vi "Step Parser.vi"(0 "Profile Step":dbl[](array[numeric]), 11 "Brushed?":bool) -> (2 "VPIpara":i32, 4 "VoltPI":dbl format="%#_13g", 6 "PPIpara":i32, 8 "PresPI":dbl format="%#_13g", 10 "CPIpara":i32, 13 "Deadhead?":bool, 15 "CmdPI":dbl format="%#_13g")   [LabVIEW 2013]
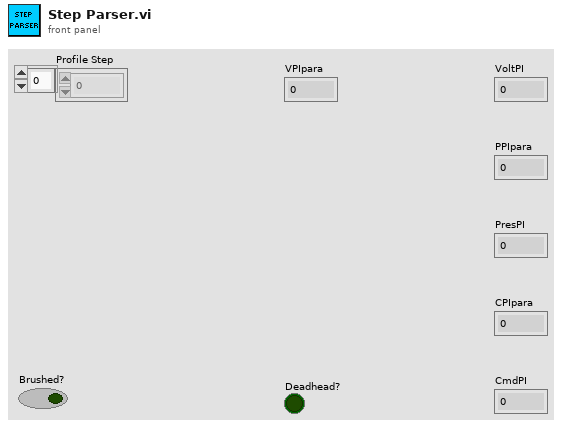
[diagram p1: front panel]
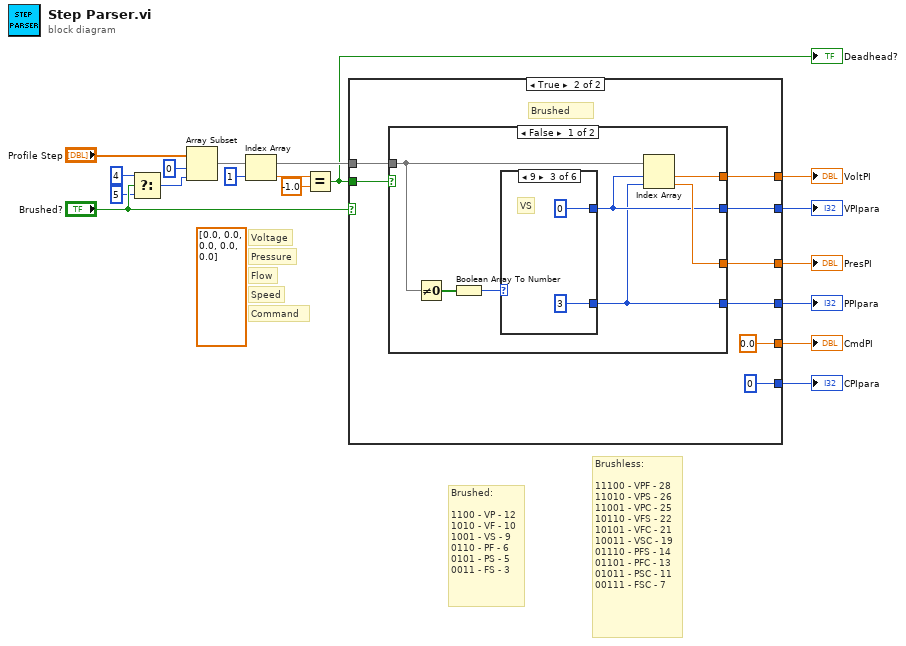
[diagram p0: block diagram]
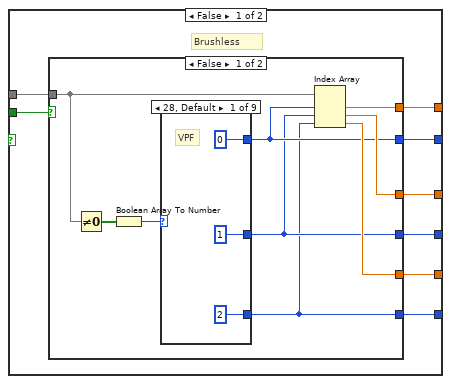
[diagram p2: hidden frame]
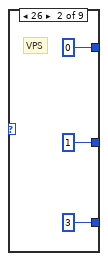
[diagram p3: hidden frame]
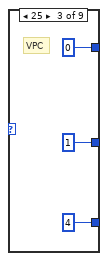
[diagram p4: hidden frame]
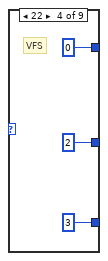
[diagram p5: hidden frame]
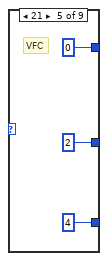
[diagram p6: hidden frame]
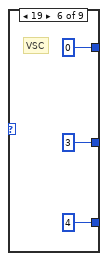
[diagram p7: hidden frame]
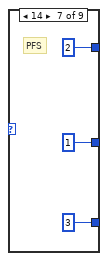
[diagram p8: hidden frame]
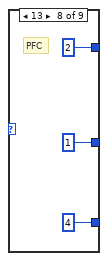
[diagram p9: hidden frame]
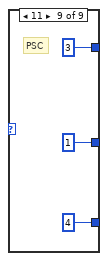
[diagram p10: hidden frame]
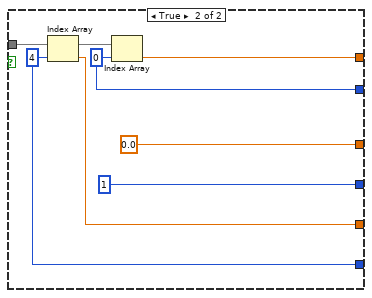
[diagram p11: hidden frame]
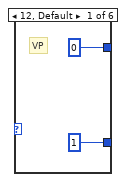
[diagram p12: hidden frame]
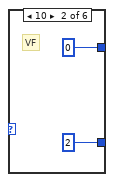
[diagram p13: hidden frame]
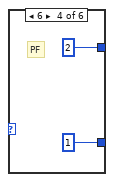
[diagram p14: hidden frame]
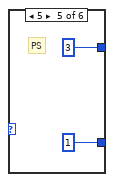
[diagram p15: hidden frame]
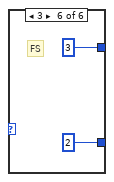
[diagram p16: hidden frame]
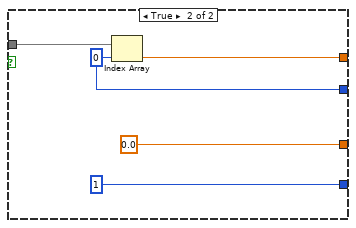
[diagram p17: hidden frame]
diagram:
  (unwired) dbl[] [0.0, 0.0, 0.0, 0.0, 0.0]
  # "Brushless:\n\n11100 - VPF - 28\n11010 - VPS - 26\n11001 - VPC - 25\n10110 - VFS - 22\n10101 - VFC - 21\n10011 - VSC - 19\n01110 - PFS - 14\n01101 - PFC - 13\n01011 - PSC - 11\n00111 - FSC - 7"
  # "Brushed:\n\n1100 - VP - 12\n1010 - VF - 10\n1001 - VS - 9\n0110 - PF - 6\n0101 - PS - 5\n0011 - FS - 3"
  # "Command"
  # "Speed"
  # "Flow"
  # "Pressure"
  # "Voltage"
  n1 = Select(t=4, s="Brushed?", f=5 ("length")) -> (s? t:f=w10:i32)
  n2 = Array Subset(array="Profile Step", index=0, length=w10) -> (w8:dbl[])
  n3 = Index Array(array=w8, index=1) -> (element=w15:dbl)
  n4 = Equal?(x=w15, y=-1.0) -> (x = y?=w7:bool)
  "Deadhead?" <- w7
  n5 = case shown="True" "Brushed?" {
    tunnel: w7 -> [w25 w73]
    tunnel: w8 -> [w24 w74]
    tunnel: [w20 0] -> w6
    tunnel: [w18 0.0] -> w5
    tunnel: [w23 w72] -> w4
    tunnel: [w22 w71] -> w3
    tunnel: [w21 w69] -> w2
    tunnel: [w19 w70] -> w1
    frame False {
      # "Brushless"
      n6 = case shown="False" w25 {
        tunnel: w24 -> [w33 w65]
        tunnel: [w31 w68] -> w23
        tunnel: [w28 w67] -> w22
        tunnel: [w27 1 ("index")] -> w21
        tunnel: [w26 w63] -> w20
        tunnel: [w30 0.0 ("element")] -> w19
        tunnel: [w29 w64] -> w18
        frame False {
          n7 = Not Equal To 0?(x=w33) -> (x != 0?=w34:bool[])
          n8 = Boolean Array To Number(Boolean array=w34) -> (number=w32:u32)
          n9 = case shown="28, Default" w32 {
            tunnel: [0 0 0 0 0 0 2 2 3] -> w28
            tunnel: [1 1 1 2 2 3 1 1 1] -> w27
            tunnel: [2 3 4 3 4 4 3 4 4] -> w26
            frame 28, Default {
              # "VPF"
            }
            frame 26 {
              # "VPS"
            }
            frame 25 {
              # "VPC"
            }
            frame 22 {
              # "VFS"
            }
            frame 21 {
              # "VFC"
            }
            frame 19 {
              # "VSC"
            }
            frame 14 {
              # "PFS"
            }
            frame 13 {
              # "PFC"
            }
            frame 11 {
              # "PSC"
            }
          }
          n10 = Index Array(array=w33, index #1=w28, index #2=w27, index #3=w26) -> (element #1=w31:dbl, element #2=w30:dbl, element #3=w29:dbl)
        }
        frame True {
          w63 = 4 ("index")
          w67 = 0 ("index")
          n11 = Index Array(array=w65, index=w63) -> (element=w64:dbl)
          n12 = Index Array(array=w65, index=w67) -> (element=w68:dbl)
        }
      }
    }
    frame True {
      # "Brushed"
      n13 = case shown="False" w73 {
        tunnel: w74 -> [w81 w97]
        tunnel: [w80 w100] -> w72
        tunnel: [w78 w99] -> w71
        tunnel: [w77 1 ("index")] -> w69
        tunnel: [w79 0.0 ("element")] -> w70
        frame False {
          n14 = Not Equal To 0?(x=w81) -> (x != 0?=w83:bool[])
          n15 = Boolean Array To Number(Boolean array=w83) -> (number=w82:u32)
          n16 = case shown="9" w82 {
            tunnel: [0 0 0 2 3 3] -> w78
            tunnel: [1 2 3 1 1 2] -> w77
            frame 12, Default {
              # "VP"
            }
            frame 10 {
              # "VF"
            }
            frame 9 {
              # "VS"
            }
            frame 6 {
              # "PF"
            }
            frame 5 {
              # "PS"
            }
            frame 3 {
              # "FS"
            }
          }
          n17 = Index Array(array=w81, index #1=w78, index #2=w77) -> (element #1=w80:dbl, element #2=w79:dbl)
        }
        frame True {
          w99 = 0 ("index")
          n18 = Index Array(array=w97, index=w99) -> (element=w100:dbl)
        }
      }
    }
  }
  "VoltPI" <- w4
  "CmdPI" <- w5
  "PresPI" <- w1
  "VPIpara" <- w3
  "PPIpara" <- w2
  "CPIpara" <- w6
